vi "SetDacValueManually_individualDAC.vi"(1 "DAC":bool, 2 "DAC write (mV)":dbl, 3 "DAC number":u8=2 min=1 max=8, 4 "RS232/ Optical Fiber":refnum<visa-resource-name>="COM2") -> (0 "DAC read (mV)":dbl)   [LabVIEW 2011]
panel:
  # "Dilution room :  COM2"
  # "Set dac value manually\nDac value is swept safely"
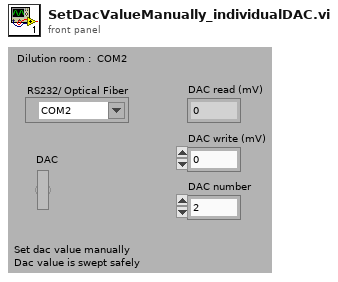
[diagram p1: front panel]
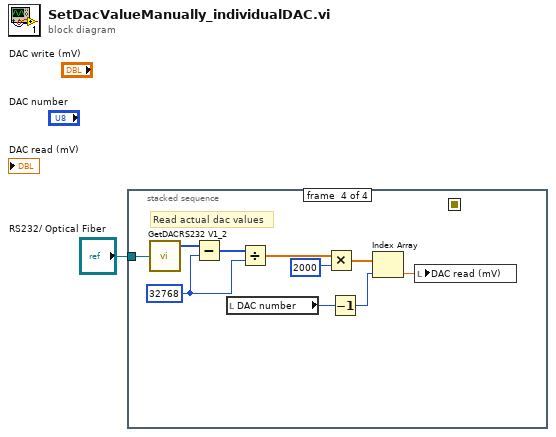
[diagram p0: block diagram]
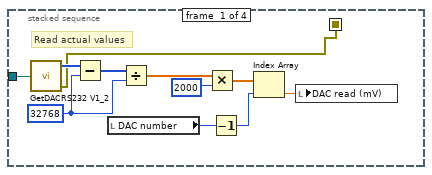
[diagram p2: hidden frame]
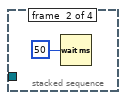
[diagram p3: hidden frame]
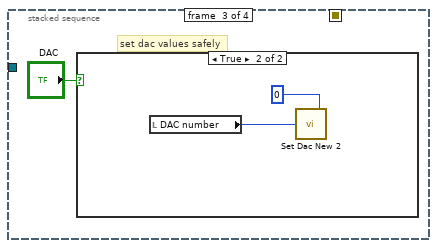
[diagram p4: hidden frame]
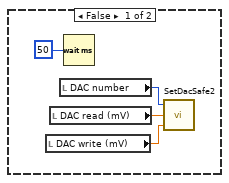
[diagram p5: hidden frame]
diagram:
  n1 = stacked-sequence {
    seq-local: [w2 _ _ _] -> [_ _ _ _]
    tunnel: "RS232/ Optical Fiber" -> [w12 _ _ w30]
    frame #0 {
      w9 = 32768
      # "Read actual values"
      n2 = call "GetDACRS232 V1_2.vi"("VISA resource name IN"=w12) -> ("error out"=w2:errorcluster, "DAC data out\n(hexadecimaal)"=w7:u16[])  [unwired: 2 in, 1 out]
      n3 = Subtract(x=w7, y=w9) -> (x-y=w8:i32[])
      n4 = local read "DAC number"() -> (w4:u8)
      n5 = Divide(x=w8, y=w9) -> (x/y=w10:dbl[])
      n6 = Multiply(x=w10, y=2000) -> (x*y=w6:dbl[])
      n7 = Decrement(x=w4) -> (x-1=w3:u8)
      n8 = Index Array(array=w6, index=w3) -> (element=w5:dbl)
      n9 = local write "DAC read (mV)"(w5) -> ()
    }
    frame #1 {
      n10 = Wait (ms)(milliseconds to wait=50) -> ()  [unwired: 1 out]
    }
    frame #2 {
      # "set dac values safely"
      n11 = case shown="True" "DAC" {
        frame False {
          n12 = local read "DAC write (mV)"() -> (w15:dbl)
          n13 = local read "DAC read (mV)"() -> (w16:dbl)
          n14 = local read "DAC number"() -> (w17:u8)
          n15 = Wait (ms)(milliseconds to wait=50) -> ()  [unwired: 1 out]
          n16 = call "SetDacSafe2.vi"("New Value (mV)"=w15, "Actual Value DAC (mV)"=w16, "DAC Nr."=w17) -> ()  [unwired: 1 out]
        }
        frame True {
          n17 = local read "DAC number"() -> (w19:u8)
          n18 = call "Set Dac New 2.vi"("DATA (V)"=0, "DAC nr"=w19) -> ()
        }
      }
    }
    frame #3 {
      w28 = 32768
      # "Read actual dac values"
      n19 = call "GetDACRS232 V1_2.vi"("VISA resource name IN"=w30) -> ("DAC data out\n(hexadecimaal)"=w26:u16[])  [unwired: 2 in, 2 out]
      n20 = Subtract(x=w26, y=w28) -> (x-y=w27:i32[])
      n21 = local read "DAC number"() -> (w22:u8)
      n22 = Divide(x=w27, y=w28) -> (x/y=w29:dbl[])
      n23 = Multiply(x=w29, y=2000) -> (x*y=w25:dbl[])
      n24 = Decrement(x=w22) -> (x-1=w21:u8)
      n25 = Index Array(array=w25, index=w21) -> (element=w24:dbl)
      n26 = local write "DAC read (mV)"(w24) -> ()
    }
  }
